vi "探头数据读取.vi"(11 "编号":string) -> ()   [LabVIEW 2016, in "斯坦道多参数.lvlib"]
panel:
  out "运行状态":u16(ring) items=["空闲", "水样测试", "标样核查"]
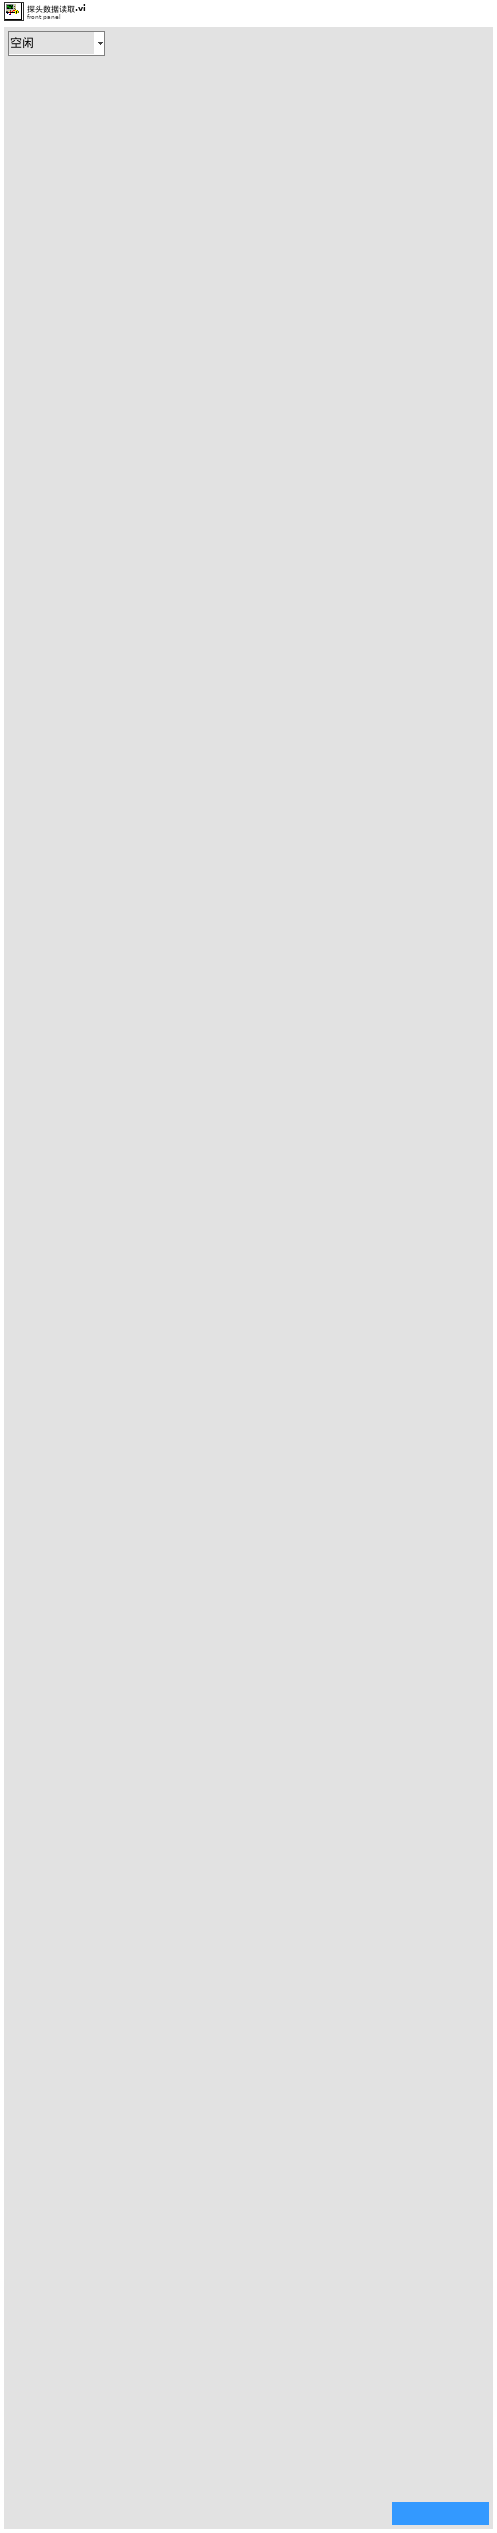
[diagram p1: front panel]
types:
  T1 = enum16{"pH", "DO", "Cond", "Turb", "ORP", "叶绿素a", "藻密度", "COD"}
  T2 = cluster{"温度测量值":sgl, "测量值":sgl, "温度偏移修正值":sgl, "信号值":sgl}
  T3 = cluster{"温度测量值":sgl, "DO%":sgl, "DOmg/L":sgl, "温度偏移修正值":sgl}
  T4 = cluster{"CH":u16, "监测值":dbl, "温度偏移修正值":sgl, "信号值":sgl}
  T5 = cluster{"pH探头选择":u16, "DO探头选择":u16, "电导率探头选择":u16, "浊度探头选择":u16, "叶绿素a探头选择":u16, "蓝绿藻探头选择":u16, "orp探头选择":u16, "COD探头选择":u16}
  T6 = cluster{"电极状态标志":u16, "电极型号标志":u16, "酸碱度测量值":sgl, "温度测量值":sgl, "酸碱度信号值":sgl, "温度信号值":sgl, "酸碱度偏移修正值":sgl, "温度偏移修正值":sgl, "手动温度补偿值":sgl, "酸碱度电极零点":sgl, "酸碱度电极斜率":sgl, "第1点标准值记录":sgl, "第1点信号值记录":sgl, "第1点温度值记录":sgl, "第2点标准值记录":sgl, "第2点信号值记录":sgl, "第2点温度值记录":sgl, "命令滤波设定":u16, "温度模式":enum16{"ATC", "MTC"}, "生产批次":u16, "电极序号":u16, "串口地址":u16, "串口波特率":enum16{"9600", "19200", "115200"}, "串口校验位":enum16{"NONE", "ODD", "EVEN"}, "串口停止位":enum16{"1bit", "2bit"}, "第一点标准值":sgl, "第二点标准值":sgl}
  T7 = cluster{"报警码":u16, "pH数值":sgl, "0X0003_NC":sgl, "温度数据":sgl, "pH原始信号 mv":sgl, "0X0009_NC":string, "产品名称":string, "序列号":string, "硬件版本":string, "软件版本":string, "通讯地址":u16, "波特率":u16, "设备类型":u16, "0X0026_NC":string, "第一点原始数据":sgl, "第一点校准数据":sgl, "第二点原始数据":sgl, "第二点校准数据":sgl, "探头校准命令":u16, "温度校准参数":sgl, "温度校准命令":u16}
  T8 = cluster{"电极状态标志":u16, "电极型号标志":u16, "电导率测量值":sgl, "温度测量值":sgl, "电导率信号值":sgl, "温度信号值":sgl, "温度补偿系数":sgl, "电导率偏移修正值":sgl, "温度偏移修正值":sgl, "手动温度补偿值":sgl, "电导率电极零点":sgl, "电导率电极斜率":sgl, "命令滤波设定":u16, "温度模式":enum16{"ATC", "MTC"}, "生产批次":u16, "电极序号":u16, "串口地址":u16, "串口波特率":enum16{"9600", "19200", "115200"}, "串口校验位":enum16{"NONE", "ODD", "EVEN"}, "串口停止位":enum16{"1bit", "2bit"}, "第一点标准值":sgl, "第二点标准值":sgl}
  T9 = cluster{"报警码":u16, "电导率数据（uS/cm）":sgl, "0x0003 NC":sgl, "温度数据":sgl, "电导率原始信号电阻":sgl, "当前量程":u16, "温度补偿系数":sgl, "0X0009_NC":string, "产品名称":string, "序列号":string, "硬件版本":string, "软件版本":string, "通讯地址":u16, "波特率":u16, "设备类型":u16, "0X0026_NC":string, "第一点原始数据":sgl, "第一点校准数据":sgl, "0X0035_NC":sgl, "0X0037_NC":sgl, "探头校准命令":u16, "温度校准参数":sgl, "温度校准命令":u16}
  T10 = cluster{"电极状态标志":u16, "电极型号标志":u16, "溶解氧测量值":sgl, "温度测量值":sgl, "溶解氧饱和度值":sgl, "盐度补偿值":sgl, "大气压补偿值":sgl, "溶解氧偏移修正值":sgl, "温度偏移修正值":sgl, "手动温度补偿值":sgl, "溶解氧电极零点":sgl, "溶解氧电极斜率":sgl, "第1点标准值记录":sgl, "第1点信号值记录":sgl, "第1点温度值记录":sgl, "第2点标准值记录":sgl, "第2点信号值记录":sgl, "第2点温度值记录":sgl, "命令滤波设定":u16, "温度模式":enum16{"ATC", "MTC"}, "生产批次":u16, "电极序号":u16, "串口地址":u16, "串口波特率":enum16{"9600", "19200", "115200"}, "串口校验位":enum16{"NONE", "ODD", "EVEN"}, "串口停止位":enum16{"1bit", "2bit"}, "第一点标准值":sgl, "第二点标准值":sgl}
  T11 = cluster{"报警码":u16, "溶解氧数值（mg/L）":sgl, "溶解氧数据（%）":sgl, "温度数据":sgl, "溶解氧原始信号 nA":sgl, "大气压力":sgl, "盐度":sgl, "0X0009_NC":string, "产品名称":string, "序列号":string, "硬件版本":string, "软件版本":string, "通讯地址":u16, "波特率":u16, "设备类型":u16, "0X0026_NC":string, "第一点原始数据":sgl, "0X0033 NC":sgl, "第二点原始数据":sgl, "0X0037 NC":sgl, "探头校准命令":u16, "温度校准参数":sgl, "温度校准命令":u16}
  T12 = cluster{"电极状态标志":u16, "电极型号标志":u16, "浊度测量值":sgl, "温度测量值":sgl, "浊度信号值":sgl, "浊度偏移修正值":sgl, "温度偏移修正值":sgl, "手动温度补偿值":sgl, "浊度电极零点":sgl, "浊度电极斜率":sgl, "第1点标准值记录":sgl, "第1点信号值记录":sgl, "第1点温度值记录":sgl, "第2点标准值记录":sgl, "第2点信号值记录":sgl, "第2点温度值记录":sgl, "命令滤波设定":u16, "温度模式":enum16{"ATC", "MTC"}, "生产批次":u16, "电极序号":u16, "串口地址":u16, "串口波特率":enum16{"9600", "19200", "115200"}, "串口校验位":enum16{"NONE", "ODD", "EVEN"}, "串口停止位":enum16{"1bit", "2bit"}, "第一点标准值":sgl, "第二点标准值":sgl, "第三点标准值":sgl}
  T13 = cluster{"报警码":u16, "浊度数值 NTU":sgl, "温度数据":sgl, "原始光强数值":u16, "量程":u16, "平均次数":u16, "清扫模式":u16, "清扫次数":u16, "清扫间隔分钟":u16, "0X000B_NC":string, "产品名称":string, "序列号":string, "硬件版本":string, "软件版本":string, "通讯地址":u16, "波特率":u16, "设备类型":u16, "0X0026_NC":string, "校准量程":u16, "第一点原始光强":u16, "第一点校准数据":sgl, "第二点原始光强":u16, "第二点校准数据":sgl, "第三点原始光强":u16, "第三点校准数据":sgl, "探头校准命令":u16, "温度校准参数":sgl, "温度校准命令":u16}
  T14 = cluster{"电极状态标志":u16, "电极型号标志":u16, "测量值":sgl, "温度测量值":sgl, "信号值":sgl, "温度信号值":sgl, "000AH_NC":sgl, "偏移修正值":sgl, "温度偏移修正值":sgl, "手动温度补偿值":sgl, "命令滤波设定":u16, "温度模式":enum16{"ATC", "MTC"}, "生产批次":u16, "传感器序号":u16, "串口地址":u16, "串口波特率":enum16{"9600", "19200", "115200"}, "串口校验位":enum16{"NONE", "ODD", "EVEN"}, "串口停止位":enum16{"1bit", "2bit"}}
  T15 = cluster{"报警码":u16, "叶绿素a":sgl, "温度数据":sgl, "原始光强数值":u16, "量程":u16, "平均次数":u16, "清扫模式":u16, "清扫次数":u16, "清扫间隔分钟":u16, "0X000B_NC":string, "产品名称":string, "序列号":string, "硬件版本":string, "软件版本":string, "通讯地址":u16, "波特率":u16, "设备类型":u16, "0X0026_NC":string, "校准量程":u16, "第一点原始光强":u16, "第一点校准数据":sgl, "第二点原始光强":u16, "第二点校准数据":sgl, "第三点原始光强":u16, "第三点校准数据":sgl, "探头校准命令":u16, "温度校准参数":sgl, "温度校准命令":u16}
  T16 = cluster{"报警码":u16, "蓝绿藻":sgl, "温度数据":sgl, "原始光强数值":u16, "0X0006_NC":u16, "平均次数":u16, "清扫模式":u16, "清扫次数":u16, "清扫间隔分钟":u16, "0X000B_NC":string, "产品名称":string, "序列号":string, "硬件版本":string, "软件版本":string, "通讯地址":u16, "波特率":u16, "设备类型":u16, "0X0026_NC":string, "0X0030_NC":u16, "第一点原始光强":u16, "第一点校准数据":sgl, "第二点原始光强":u16, "第二点校准数据":sgl, "第三点原始光强":u16, "第三点校准数据":sgl, "探头校准命令":u16, "温度校准参数":sgl, "温度校准命令":u16}
  T17 = cluster{"电极状态标志":u16, "电极型号标志":u16, "COD测量值":sgl, "浊度测量值":sgl, "COD信号值":sgl, "浊度信号值":sgl, "温度测量值":sgl, "COD偏移修正值":sgl, "浊度偏移修正值":sgl, "COD水样校正值":sgl, "温度偏移修正值":sgl, "COD零点系数":sgl, "COD斜率系数":sgl, "浊度零点系数":sgl, "浊度斜率系数":sgl, "COD测值K值":sgl, "浊度测值K值":sgl, "浊度补偿COD系数值":sgl, "COD温度补偿系数值 ":sgl, "测量周期":u16, "清洗周期":u16, "命令寄存器":u16, "数字滤波设定":u16, "温度模式":enum16{"AUTO", "OFF"}, "生产批次":u16, "电极序号":u16, "串口地址":u16, "串口波特率":enum16{"9600", "19200", "115200"}, "串口校验位":enum16{"NONE", "ODD", "EVEN"}, "串口停止位":enum16{"1bit", "2bit"}, "第一点校正指令":u16, "第一点标准值":sgl, "第二点校正指令":u16, "第二点标准值":sgl, "第三点校正指令":u16, "第三点标准值":sgl, "COD吸光度":sgl, "浊度吸光度":sgl, "温度信号值":sgl}
  T18 = enum16{"pH", "DO", "Cond", "Turb", "ORP", "叶绿素a", "藻密度", "COD"}[]
  T19 = cluster{"ph":bool, "DO":bool, "Cond":bool, "Turb":bool, "叶绿素a":bool, "藻密度":bool, "ORP":bool, "COD":bool}
  T20 = cluster{"ph":bool, "DO":bool, "Cond":bool, "Turb":bool, "叶绿素a":bool, "藻密度":bool, "ORP":bool, "cod":bool}
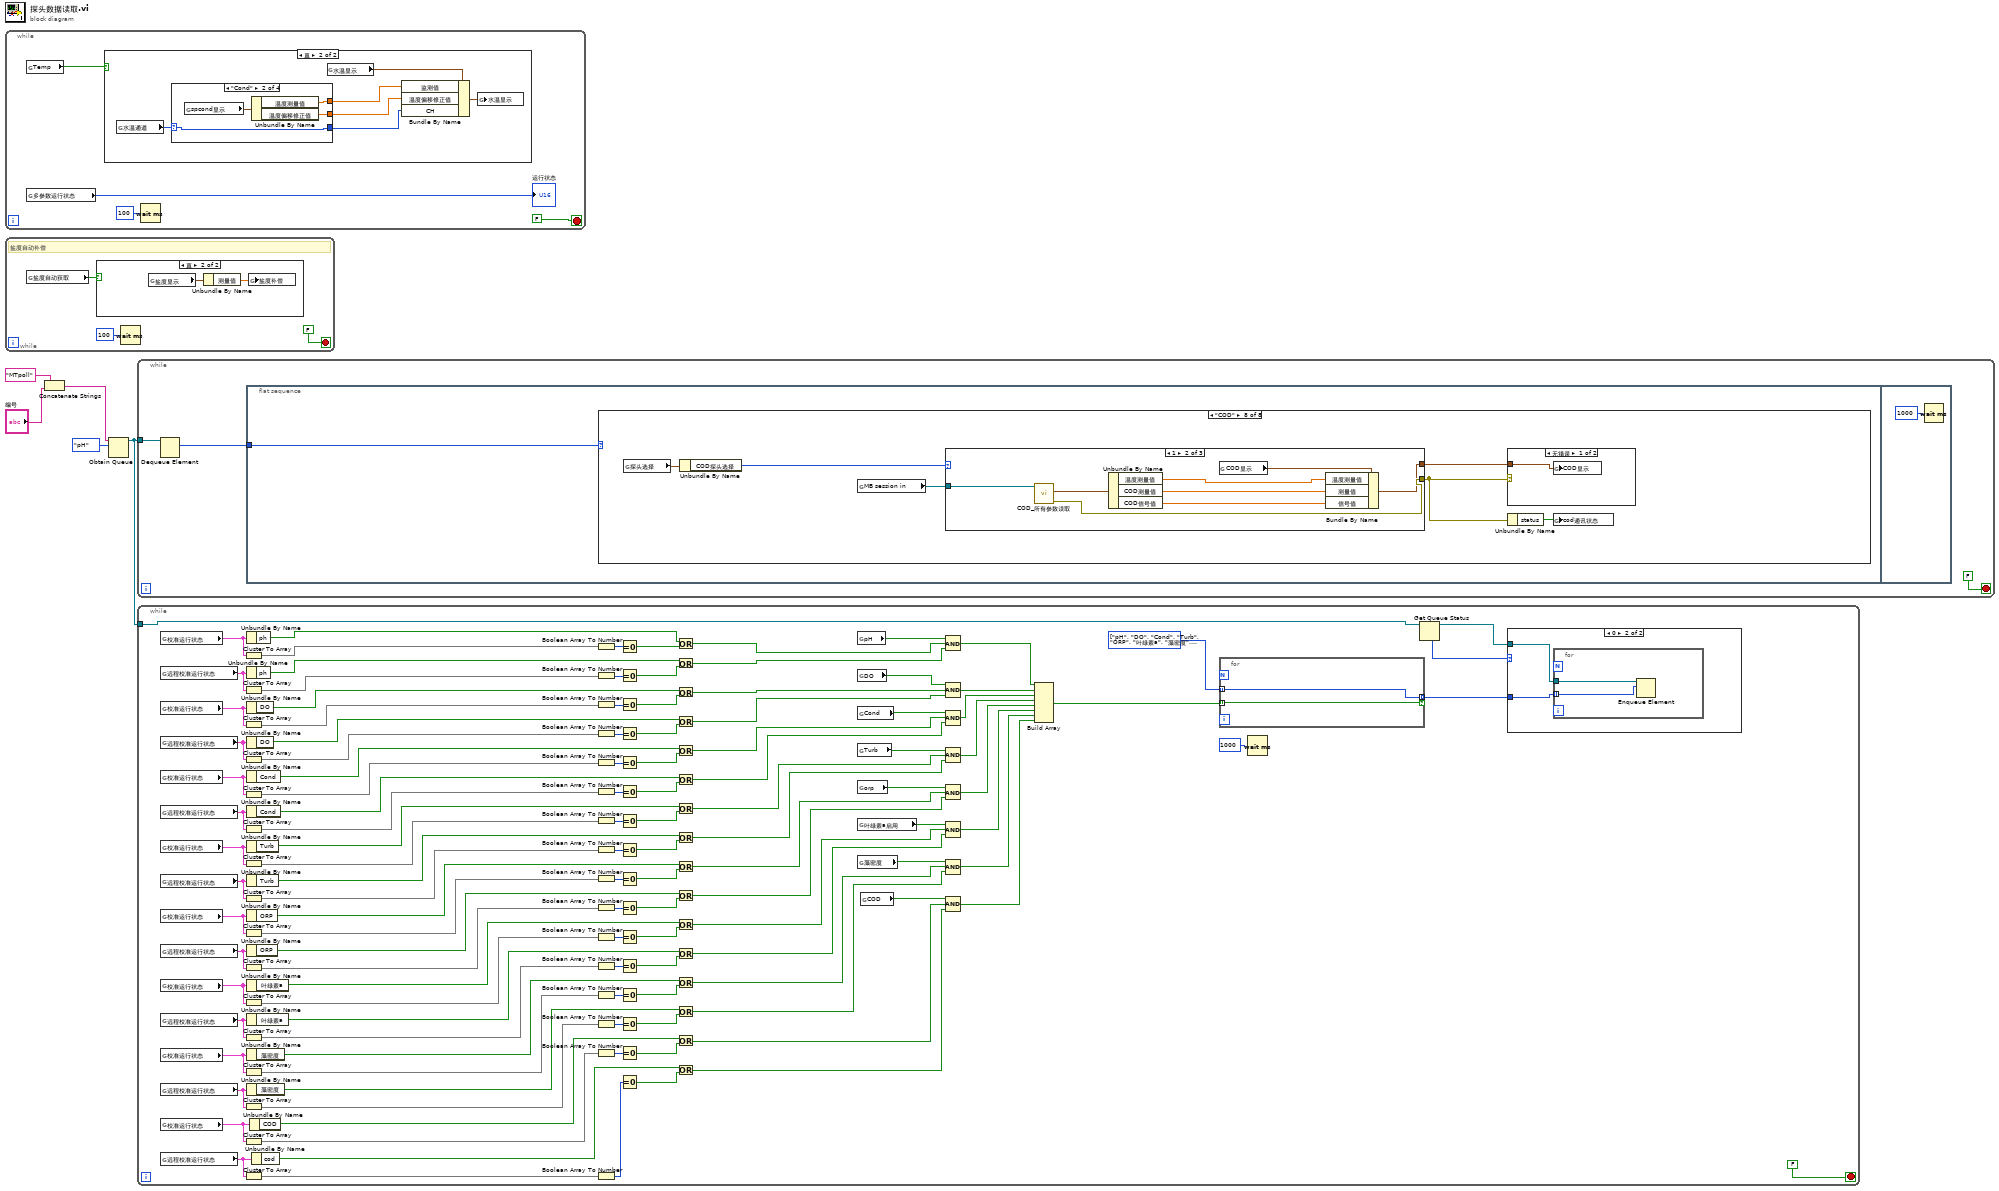
[diagram p0: block diagram]
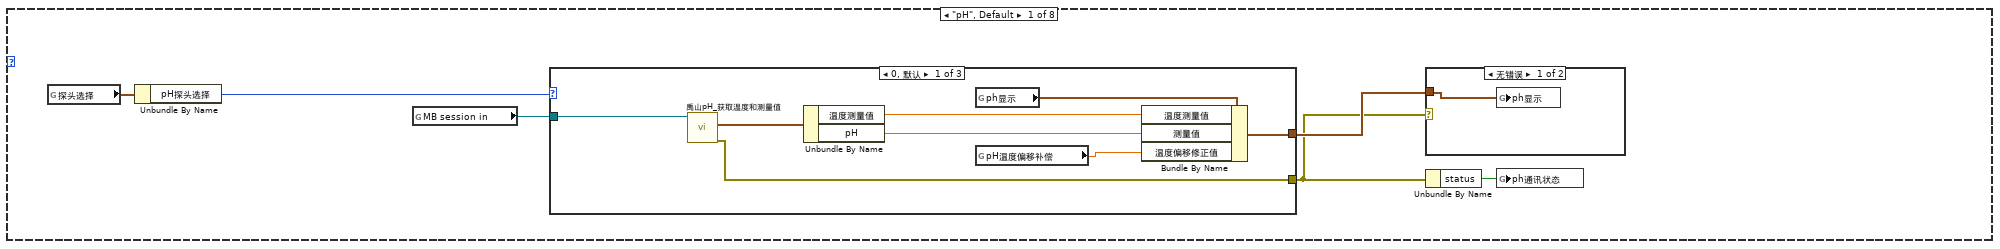
[diagram p3: hidden frame]
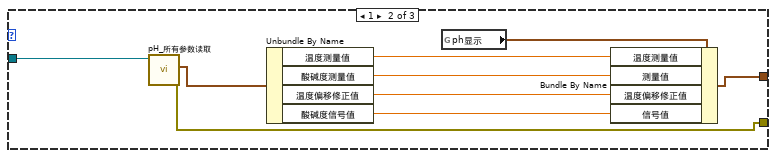
[diagram p4: hidden frame]
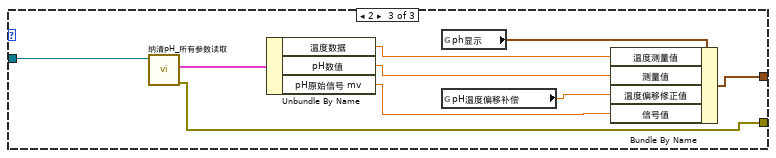
[diagram p5: hidden frame]
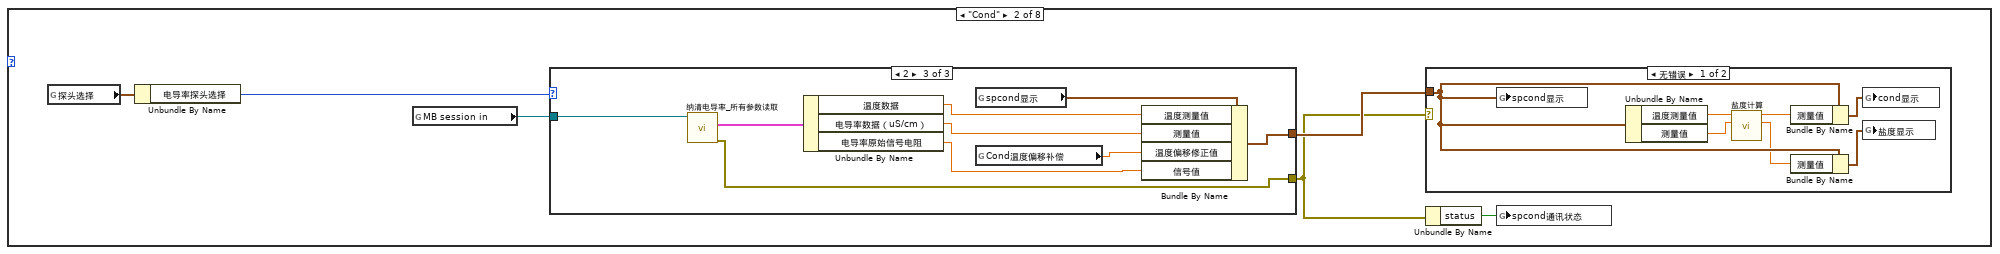
[diagram p7: hidden frame]
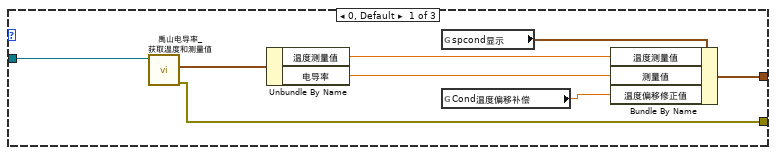
[diagram p8: hidden frame]
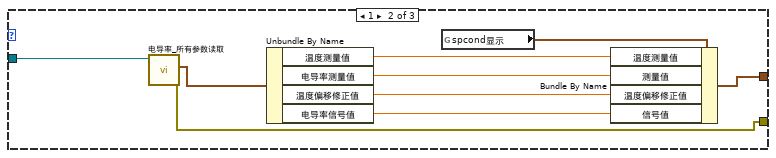
[diagram p9: hidden frame]
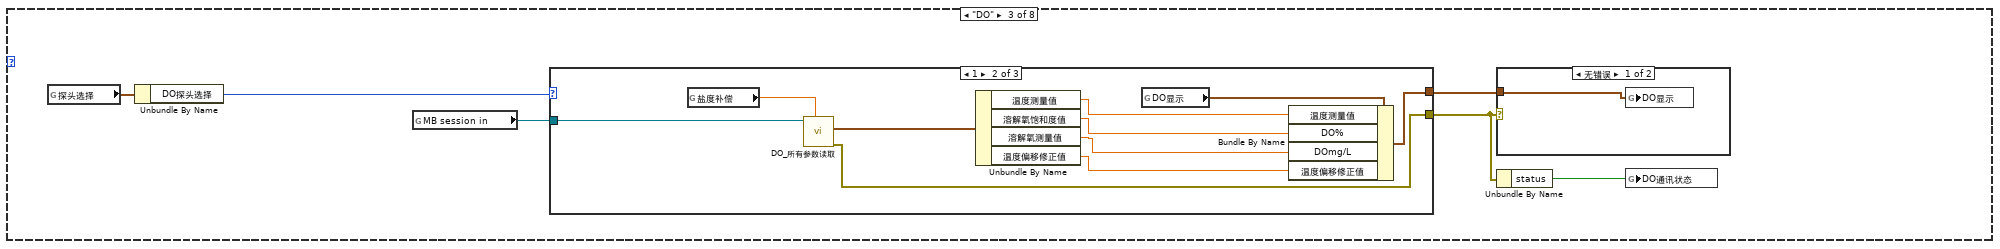
[diagram p11: hidden frame]
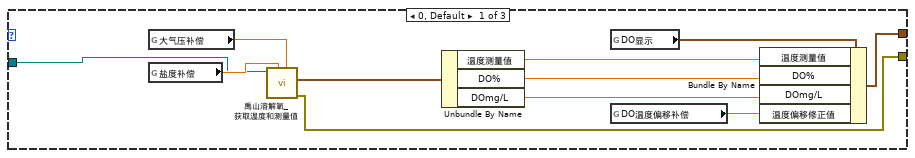
[diagram p12: hidden frame]
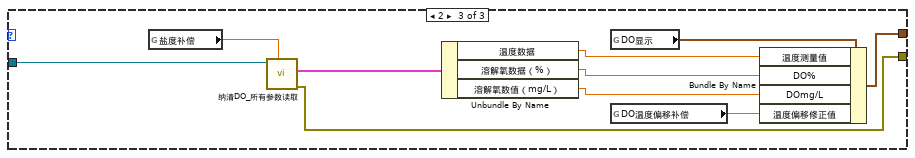
[diagram p13: hidden frame]
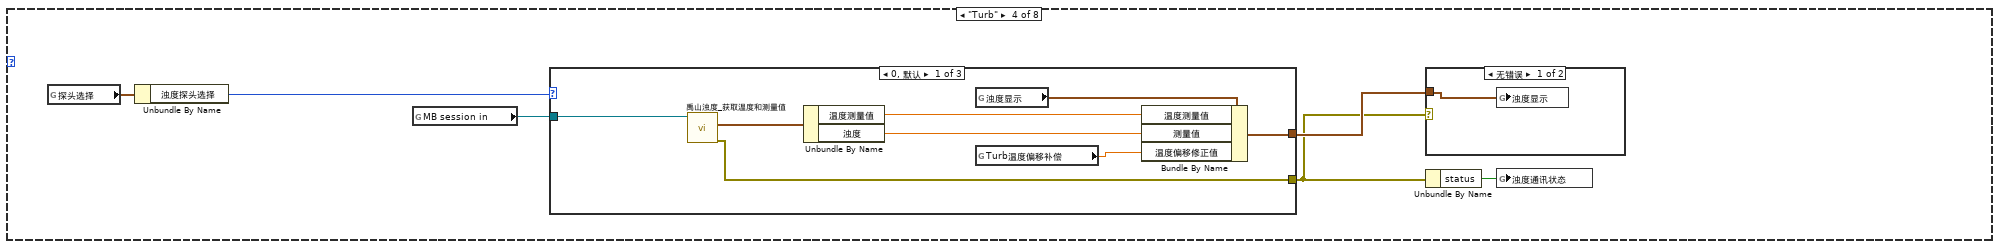
[diagram p15: hidden frame]
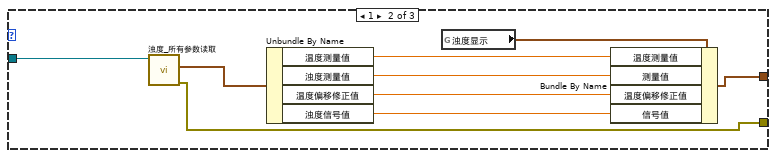
[diagram p16: hidden frame]
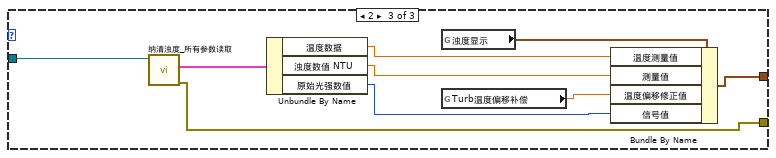
[diagram p17: hidden frame]
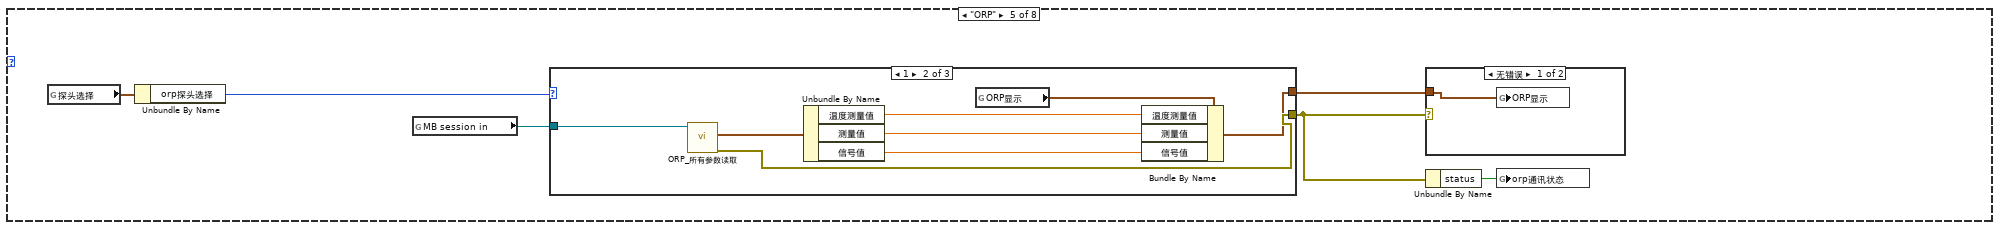
[diagram p19: hidden frame]
diagram:
  n1 = while {
    stop <- FALSE stop-if-true
    n2 = global read "断电保存变量.vi" "Temp"() -> (w7:bool)
    n3 = global read "多参数全局变量.vi" "多参数运行状态"() -> (→"运行状态":u16)
    n4 = case shown="真" w7 {
      frame False {
      }
      frame True {
        n5 = global read "断电保存变量.vi" "水温通道"() -> (w15:enum16{"pH", "Cond", "DO", "Turb"})
        n6 = case shown="\"Cond\"" w15 {
          selector: w15 -> [w19 w23 w27 w31]
          tunnel: [w19 w23 w27 w31] -> w14
          tunnel: [w17 w20 w24 w28] -> w13
          tunnel: [w18 w21 w25 w29] -> w12
          frame "pH", Default {
            n7 = global read "多参数全局变量.vi" "ph显示"() -> (w16:T2)
            n8 = Unbundle By Name(w16) -> ("温度测量值"=w18:sgl, "温度偏移修正值"=w17:sgl)
          }
          frame "Cond" {
            n9 = global read "多参数全局变量.vi" "spcond显示"() -> (w22:T2)
            n10 = Unbundle By Name(w22) -> ("温度测量值"=w21:sgl, "温度偏移修正值"=w20:sgl)
          }
          frame "DO" {
            n11 = global read "多参数全局变量.vi" "DO显示"() -> (w26:T3)
            n12 = Unbundle By Name(w26) -> ("温度测量值"=w25:sgl, "温度偏移修正值"=w24:sgl)
          }
          frame "Turb" {
            n13 = global read "多参数全局变量.vi" "浊度显示"() -> (w30:T2)
            n14 = Unbundle By Name(w30) -> ("温度测量值"=w29:sgl, "温度偏移修正值"=w28:sgl)
          }
        }
        n15 = global read "多参数全局变量.vi" "水温显示"() -> (w10:T4)
        n16 = Bundle By Name(cluster=w10, "监测值"=w12, "温度偏移修正值"=w13, "CH"=w14) -> (w11:T4)
        n17 = global write "多参数全局变量.vi" "水温显示"(w11) -> ()
      }
    }
    n18 = Wait (ms)(milliseconds to wait=u32 100 ("等待时间（毫秒）")) -> ()  [unwired: 1 out]
  }
  n19 = while {
    stop <- FALSE stop-if-true
    # "盐度自动补偿"
    n20 = global read "断电保存变量.vi" "盐度自动获取"() -> (w33:bool)
    n21 = case shown="真" w33 {
      frame False {
      }
      frame True {
        n22 = global read "多参数全局变量.vi" "盐度显示"() -> (w36:T2)
        n23 = Unbundle By Name(w36) -> ("测量值"=w35:sgl)
        n24 = global write "断电保存变量.vi" "盐度补偿"(w35) -> ()
      }
    }
    n25 = Wait (ms)(milliseconds to wait=u32 100 ("等待时间（毫秒）")) -> ()  [unwired: 1 out]
  }
  n26 = Concatenate Strings("MTpoll" ("名称（未命名）"), "编号") -> (w3:string)
  n27 = Obtain Queue(name (unnamed)=w3, element data type=T1."pH" ("枚举")) -> (queue out=w1:refnum<queue>)  [unwired: 3 in, 2 out]
  n28 = while {
    tunnel: w1 -> [w39]
    stop <- FALSE stop-if-true
    n29 = Dequeue Element(queue=w39) -> (element=w38:T1)  [unwired: 2 in, 3 out]
    n30 = flat-sequence {
      tunnel: w38 -> [w40]
      frame #0 {
        n31 = case shown="\"COD\"" w40 {
          frame "pH", Default {
            n32 = global read "断电保存变量.vi" "探头选择"() -> (w46:T5)
            n33 = Unbundle By Name(w46) -> ("pH探头选择"=w45:u16)
            n34 = global read "多参数全局变量.vi" "MB session in"() -> (w44:refnum<class "MB_Master.lvclass">)
            n35 = case shown="0, 默认" w45 {
              tunnel: w44 -> [w54 w63 w70]
              tunnel: [w53 w62 w68] -> w42
              tunnel: [w51 w59 w71] -> w43
              frame 0, Default {
                n36 = call "禹山pH_获取温度和测量值.vi"("MB session in"=w54) -> ("error out"=w53:errorcluster, "输出值"=w50:cluster{"温度测量值":sgl, "ORP":sgl, "pH":sgl})  [unwired: 8 in, 1 out]
                n37 = Unbundle By Name(w50) -> ("温度测量值"=w49:sgl, "pH"=w48:sgl)
                n38 = global read "多参数全局变量.vi" "ph显示"() -> (w52:T2)
                n39 = global read "断电保存变量.vi" "pH温度偏移补偿"() -> (w47:dbl)
                n40 = Bundle By Name(cluster=w52, "温度测量值"=w49, "测量值"=w48, "温度偏移修正值"=w47) -> (w51:T2)
              }
              frame 1 {
                n41 = call "pH_所有参数读取.vi"("MB session in"=w63) -> ("error out"=w62:errorcluster, "输出值"=w61:T6)  [unwired: 8 in, 1 out]
                n42 = Unbundle By Name(w61) -> ("温度测量值"=w56:sgl, "酸碱度测量值"=w57:sgl, "温度偏移修正值"=w58:sgl, "酸碱度信号值"=w55:sgl)
                n43 = global read "多参数全局变量.vi" "ph显示"() -> (w60:T2)
                n44 = Bundle By Name(cluster=w60, "温度测量值"=w56, "测量值"=w57, "温度偏移修正值"=w58, "信号值"=w55) -> (w59:T2)
              }
              frame 2 {
                n45 = call "纳清pH_所有参数读取.vi"("MB session in"=w70) -> ("error out"=w68:errorcluster, "输出值"=w69:T7)  [unwired: 8 in, 1 out]
                n46 = Unbundle By Name(w69) -> ("温度数据"=w67:sgl, "pH数值"=w66:sgl, "pH原始信号 mv"=w64:sgl)
                n47 = global read "多参数全局变量.vi" "ph显示"() -> (w72:T2)
                n48 = global read "断电保存变量.vi" "pH温度偏移补偿"() -> (w65:dbl)
                n49 = Bundle By Name(cluster=w72, "温度测量值"=w67, "测量值"=w66, "温度偏移修正值"=w65, "信号值"=w64) -> (w71:T2)
              }
            }
            n50 = case shown="无错误" w42 {
              tunnel: w43 -> [w73 _]
              frame No Error {
                n51 = global write "多参数全局变量.vi" "ph显示"(w73) -> ()
              }
              frame Error {
              }
            }
            n52 = Unbundle By Name(w42) -> ("status"=w41:bool)
            n53 = global write "多参数全局变量.vi" "ph通讯状态"(w41) -> ()
          }
          frame "Cond" {
            n54 = global read "断电保存变量.vi" "探头选择"() -> (w79:T5)
            n55 = Unbundle By Name(w79) -> ("电导率探头选择"=w78:u16)
            n56 = global read "多参数全局变量.vi" "MB session in"() -> (w76:refnum<class "MB_Master.lvclass">)
            n57 = case shown="2" w78 {
              tunnel: w76 -> [w87 w96 w101]
              tunnel: [w81 w94 w104] -> w77
              tunnel: [w86 w93 w99] -> w75
              frame 0, Default {
                n58 = call "禹山电导率_获取温度和测量值.vi"("MB session in"=w87) -> ("error out"=w86:errorcluster, "输出值"=w84:cluster{"温度测量值":sgl, "电导率":sgl, "错误标志":u16})  [unwired: 8 in, 1 out]
                n59 = Unbundle By Name(w84) -> ("温度测量值"=w83:sgl, "电导率"=w82:sgl)
                n60 = global read "多参数全局变量.vi" "spcond显示"() -> (w85:T2)
                n61 = global read "断电保存变量.vi" "Cond温度偏移补偿"() -> (w80:dbl)
                n62 = Bundle By Name(cluster=w85, "温度测量值"=w83, "测量值"=w82, "温度偏移修正值"=w80) -> (w81:T2)
              }
              frame 1 {
                n63 = call "电导率_所有参数读取.vi"("MB session in"=w96) -> ("error out"=w93:errorcluster, "输出值"=w92:T8)  [unwired: 8 in, 1 out]
                n64 = Unbundle By Name(w92) -> ("温度测量值"=w91:sgl, "电导率测量值"=w90:sgl, "温度偏移修正值"=w89:sgl, "电导率信号值"=w88:sgl)
                n65 = global read "多参数全局变量.vi" "spcond显示"() -> (w95:T2)
                n66 = Bundle By Name(cluster=w95, "温度测量值"=w91, "测量值"=w90, "温度偏移修正值"=w89, "信号值"=w88) -> (w94:T2)
              }
              frame 2 {
                n67 = call "纳清电导率_所有参数读取.vi"("MB session in"=w101) -> ("error out"=w99:errorcluster, "输出值"=w100:T9)  [unwired: 8 in, 1 out]
                n68 = Unbundle By Name(w100) -> ("温度数据"=w103:sgl, "电导率数据（uS/cm）"=w102:sgl, "电导率原始信号电阻"=w97:sgl)
                n69 = global read "多参数全局变量.vi" "spcond显示"() -> (w105:T2)
                n70 = global read "断电保存变量.vi" "Cond温度偏移补偿"() -> (w98:dbl)
                n71 = Bundle By Name(cluster=w105, "温度测量值"=w103, "测量值"=w102, "温度偏移修正值"=w98, "信号值"=w97) -> (w104:T2)
              }
            }
            n72 = case shown="无错误" w75 {
              tunnel: w77 -> [w107 _]
              frame No Error {
                n73 = global write "多参数全局变量.vi" "spcond显示"(w107) -> ()
                n74 = Unbundle By Name(w107) -> ("温度测量值"=w112:sgl, "测量值"=w111:sgl)
                n75 = call "盐度计算.vi"("spCond"=w111, "Temp"=w112) -> ("saltresult"=w106:dbl, "cond"=w110:dbl)  [unwired: 8 in]
                n76 = Bundle By Name(cluster=w107, "测量值"=w110) -> (w109:T2)
                n77 = Bundle By Name(cluster=w107, "测量值"=w106) -> (w108:T2)
                n78 = global write "多参数全局变量.vi" "cond显示"(w109) -> ()
                n79 = global write "多参数全局变量.vi" "盐度显示"(w108) -> ()
              }
              frame Error {
              }
            }
            n80 = Unbundle By Name(w75) -> ("status"=w74:bool)
            n81 = global write "多参数全局变量.vi" "spcond通讯状态"(w74) -> ()
          }
          frame "DO" {
            n82 = global read "断电保存变量.vi" "探头选择"() -> (w118:T5)
            n83 = Unbundle By Name(w118) -> ("DO探头选择"=w117:u16)
            n84 = global read "多参数全局变量.vi" "MB session in"() -> (w115:refnum<class "MB_Master.lvclass">)
            n85 = case shown="1" w117 {
              tunnel: w115 -> [w127 w139 w144]
              tunnel: [w125 w137 w148] -> w116
              tunnel: [w121 w132 w142] -> w114
              frame 0, Default {
                n86 = global read "断电保存变量.vi" "大气压补偿"() -> (w128:dbl)
                n87 = global read "断电保存变量.vi" "盐度补偿"() -> (w129:dbl)
                n88 = call "禹山溶解氧_获取温度和测量值.vi"("大气压补偿"=w128, "盐度补偿"=w129, "MB session in"=w127) -> ("error out"=w121:errorcluster, "输出值"=w119:cluster{"温度测量值":sgl, "DO%":sgl, "DOmg/L":sgl})  [unwired: 6 in, 1 out]
                n89 = Unbundle By Name(w119) -> ("温度测量值"=w124:sgl, "DO%"=w123:sgl, "DOmg/L"=w122:sgl)
                n90 = global read "多参数全局变量.vi" "DO显示"() -> (w126:T3)
                n91 = global read "断电保存变量.vi" "DO温度偏移补偿"() -> (w120:dbl)
                n92 = Bundle By Name(cluster=w126, "温度测量值"=w124, "DO%"=w123, "DOmg/L"=w122, "温度偏移修正值"=w120) -> (w125:T3)
              }
              frame 1 {
                n93 = global read "断电保存变量.vi" "盐度补偿"() -> (w130:dbl)
                n94 = call "DO_所有参数读取.vi"("盐度补偿"=w130, "MB session in"=w139) -> ("error out"=w132:errorcluster, "输出值"=w136:T10)  [unwired: 7 in, 1 out]
                n95 = Unbundle By Name(w136) -> ("温度测量值"=w133:sgl, "溶解氧饱和度值"=w134:sgl, "溶解氧测量值"=w135:sgl, "温度偏移修正值"=w131:sgl)
                n96 = global read "多参数全局变量.vi" "DO显示"() -> (w138:T3)
                n97 = Bundle By Name(cluster=w138, "温度测量值"=w133, "DO%"=w134, "DOmg/L"=w135, "温度偏移修正值"=w131) -> (w137:T3)
              }
              frame 2 {
                n98 = global read "断电保存变量.vi" "盐度补偿"() -> (w140:dbl)
                n99 = call "纳清DO_所有参数读取.vi"("盐度补偿"=w140, "MB session in"=w144) -> ("error out"=w142:errorcluster, "输出值"=w143:T11)  [unwired: 7 in, 1 out]
                n100 = Unbundle By Name(w143) -> ("温度数据"=w145:sgl, "溶解氧数据（%）"=w146:sgl, "溶解氧数值（mg/L）"=w147:sgl)
                n101 = global read "多参数全局变量.vi" "DO显示"() -> (w149:T3)
                n102 = global read "断电保存变量.vi" "DO温度偏移补偿"() -> (w141:dbl)
                n103 = Bundle By Name(cluster=w149, "温度测量值"=w145, "DO%"=w146, "DOmg/L"=w147, "温度偏移修正值"=w141) -> (w148:T3)
              }
            }
            n104 = case shown="无错误" w114 {
              tunnel: w116 -> [w150 _]
              frame No Error {
                n105 = global write "多参数全局变量.vi" "DO显示"(w150) -> ()
              }
              frame Error {
              }
            }
            n106 = Unbundle By Name(w114) -> ("status"=w113:bool)
            n107 = global write "多参数全局变量.vi" "DO通讯状态"(w113) -> ()
          }
          frame "Turb" {
            n108 = global read "断电保存变量.vi" "探头选择"() -> (w156:T5)
            n109 = Unbundle By Name(w156) -> ("浊度探头选择"=w155:u16)
            n110 = global read "多参数全局变量.vi" "MB session in"() -> (w153:refnum<class "MB_Master.lvclass">)
            n111 = case shown="0, 默认" w155 {
              tunnel: w153 -> [w164 w173 w178]
              tunnel: [w162 w168 w179] -> w154
              tunnel: [w161 w167 w177] -> w152
              frame 0, Default {
                n112 = call "禹山浊度_获取温度和测量值.vi"("MB session in"=w164) -> ("error out"=w161:errorcluster, "输出值"=w160:cluster{"温度测量值":sgl, "浊度":sgl})  [unwired: 8 in, 1 out]
                n113 = Unbundle By Name(w160) -> ("温度测量值"=w159:sgl, "浊度"=w158:sgl)
                n114 = global read "多参数全局变量.vi" "浊度显示"() -> (w163:T2)
                n115 = global read "断电保存变量.vi" "Turb温度偏移补偿"() -> (w157:dbl)
                n116 = Bundle By Name(cluster=w163, "温度测量值"=w159, "测量值"=w158, "温度偏移修正值"=w157) -> (w162:T2)
              }
              frame 1 {
                n117 = call "浊度_所有参数读取.vi"("MB session in"=w173) -> ("error out"=w167:errorcluster, "输出值"=w172:T12)  [unwired: 8 in, 1 out]
                n118 = Unbundle By Name(w172) -> ("温度测量值"=w170:sgl, "浊度测量值"=w169:sgl, "温度偏移修正值"=w166:sgl, "浊度信号值"=w165:sgl)
                n119 = global read "多参数全局变量.vi" "浊度显示"() -> (w171:T2)
                n120 = Bundle By Name(cluster=w171, "温度测量值"=w170, "测量值"=w169, "温度偏移修正值"=w166, "信号值"=w165) -> (w168:T2)
              }
              frame 2 {
                n121 = call "纳清浊度_所有参数读取.vi"("MB session in"=w178) -> ("error out"=w177:errorcluster, "输出值"=w176:T13)  [unwired: 8 in, 1 out]
                n122 = Unbundle By Name(w176) -> ("温度数据"=w181:sgl, "浊度数值 NTU"=w180:sgl, "原始光强数值"=w174:u16)
                n123 = global read "多参数全局变量.vi" "浊度显示"() -> (w182:T2)
                n124 = global read "断电保存变量.vi" "Turb温度偏移补偿"() -> (w175:dbl)
                n125 = Bundle By Name(cluster=w182, "温度测量值"=w181, "测量值"=w180, "温度偏移修正值"=w175, "信号值"=w174) -> (w179:T2)
              }
            }
            n126 = case shown="无错误" w152 {
              tunnel: w154 -> [w183 _]
              frame No Error {
                n127 = global write "多参数全局变量.vi" "浊度显示"(w183) -> ()
              }
              frame Error {
              }
            }
            n128 = Unbundle By Name(w152) -> ("status"=w151:bool)
            n129 = global write "多参数全局变量.vi" "浊度通讯状态"(w151) -> ()
          }
          frame "ORP" {
            n130 = global read "断电保存变量.vi" "探头选择"() -> (w188:T5)
            n131 = Unbundle By Name(w188) -> ("orp探头选择"=w187:u16)
            n132 = global read "多参数全局变量.vi" "MB session in"() -> (w186:refnum<class "MB_Master.lvclass">)
            n133 = case shown="1" w187 {
              tunnel: [_ w192 _] -> w185
              tunnel: w186 -> [_ w197 _]
              tunnel: [_ w190 _] -> w189
              frame 0, Default {
              }
              frame 1 {
                n134 = call "ORP_所有参数读取.vi"("MB session in"=w197) -> ("error out"=w192:errorcluster, "输出值"=w194:T14)  [unwired: 8 in, 1 out]
                n135 = Unbundle By Name(w194) -> ("温度测量值"=w195:sgl, "测量值"=w196:sgl, "信号值"=w191:sgl)
                n136 = global read "多参数全局变量.vi" "ORP显示"() -> (w193:T2)
                n137 = Bundle By Name(cluster=w193, "温度测量值"=w195, "测量值"=w196, "信号值"=w191) -> (w190:T2)
              }
              frame 2 {
              }
            }
            n138 = case shown="无错误" w185 {
              tunnel: w189 -> [w198 _]
              frame No Error {
                n139 = global write "多参数全局变量.vi" "ORP显示"(w198) -> ()
              }
              frame Error {
              }
            }
            n140 = Unbundle By Name(w185) -> ("status"=w184:bool)
            n141 = global write "多参数全局变量.vi" "orp通讯状态"(w184) -> ()
          }
          frame "叶绿素a" {
            n142 = global read "断电保存变量.vi" "探头选择"() -> (w203:T5)
            n143 = Unbundle By Name(w203) -> ("叶绿素a探头选择"=w202:u16)
            n144 = global read "多参数全局变量.vi" "MB session in"() -> (w201:refnum<class "MB_Master.lvclass">)
            n145 = case shown="2" w202 {
              tunnel: [w211 _ w217] -> w200
              tunnel: w201 -> [w210 _ w219]
              tunnel: [w208 _ w216] -> w204
              frame 0, Default {
                n146 = call "叶绿素a_获取温度和叶绿素值.vi"("MB session in"=w210) -> ("error out"=w211:errorcluster, "输出值"=w207:cluster{"温度测量值":sgl, "叶绿素测量值":sgl, "错误标志":u16})  [unwired: 8 in, 1 out]
                n147 = Unbundle By Name(w207) -> ("温度测量值"=w205:sgl, "叶绿素测量值"=w206:sgl)
                n148 = global read "多参数全局变量.vi" "叶绿素a显示"() -> (w209:T2)
                n149 = Bundle By Name(cluster=w209, "温度测量值"=w205, "测量值"=w206) -> (w208:T2)
              }
              frame 1 {
              }
              frame 2 {
                n150 = call "纳清叶绿素a_所有参数读取.vi"("MB session in"=w219) -> ("error out"=w217:errorcluster, "输出值"=w215:T15)  [unwired: 8 in, 1 out]
                n151 = Unbundle By Name(w215) -> ("温度数据"=w213:sgl, "叶绿素a"=w214:sgl, "原始光强数值"=w212:u16)
                n152 = global read "多参数全局变量.vi" "叶绿素a显示"() -> (w218:T2)
                n153 = Bundle By Name(cluster=w218, "温度测量值"=w213, "测量值"=w214, "信号值"=w212) -> (w216:T2)
              }
            }
            n154 = case shown="无错误" w200 {
              tunnel: w204 -> [w220 _]
              frame No Error {
                n155 = global write "多参数全局变量.vi" "叶绿素a显示"(w220) -> ()
              }
              frame Error {
              }
            }
            n156 = Unbundle By Name(w200) -> ("status"=w199:bool)
            n157 = global write "多参数全局变量.vi" "叶绿素a通讯状态"(w199) -> ()
          }
          frame "藻密度" {
            n158 = global read "断电保存变量.vi" "探头选择"() -> (w225:T5)
            n159 = Unbundle By Name(w225) -> ("蓝绿藻探头选择"=w224:u16)
            n160 = global read "多参数全局变量.vi" "MB session in"() -> (w223:refnum<class "MB_Master.lvclass">)
            n161 = case shown="2" w224 {
              tunnel: [_ _ w232] -> w222
              tunnel: w223 -> [_ _ w234]
              tunnel: [_ _ w231] -> w226
              frame 0, Default {
              }
              frame 1 {
              }
              frame 2 {
                n162 = call "纳清蓝绿藻_所有参数读取.vi"("MB session in"=w234) -> ("error out"=w232:errorcluster, "输出值"=w230:T16)  [unwired: 8 in, 1 out]
                n163 = Unbundle By Name(w230) -> ("温度数据"=w229:sgl, "蓝绿藻"=w228:sgl, "原始光强数值"=w227:u16)
                n164 = global read "多参数全局变量.vi" "藻密度显示"() -> (w233:T2)
                n165 = Bundle By Name(cluster=w233, "温度测量值"=w229, "测量值"=w228, "信号值"=w227) -> (w231:T2)
              }
            }
            n166 = case shown="无错误" w222 {
              tunnel: w226 -> [w235 _]
              frame No Error {
                n167 = global write "多参数全局变量.vi" "藻密度显示"(w235) -> ()
              }
              frame Error {
              }
            }
            n168 = Unbundle By Name(w222) -> ("status"=w221:bool)
            n169 = global write "多参数全局变量.vi" "藻密度通讯状态"(w221) -> ()
          }
          frame "COD" {
            n170 = global read "断电保存变量.vi" "探头选择"() -> (w240:T5)
            n171 = Unbundle By Name(w240) -> ("COD探头选择"=w239:u16)
            n172 = global read "多参数全局变量.vi" "MB session in"() -> (w238:refnum<class "MB_Master.lvclass">)
            n173 = case shown="1" w239 {
              tunnel: [_ w247 _] -> w237
              tunnel: w238 -> [_ w249 _]
              tunnel: [_ w246 _] -> w241
              frame 0, Default {
              }
              frame 1 {
                n174 = call "COD_所有参数读取.vi"("MB session in"=w249) -> ("error out"=w247:errorcluster, "输出值"=w245:T17)  [unwired: 8 in, 1 out]
                n175 = Unbundle By Name(w245) -> ("温度测量值"=w244:sgl, "COD测量值"=w243:sgl, "COD信号值"=w242:sgl)
                n176 = global read "多参数全局变量.vi" "COD显示"() -> (w248:T2)
                n177 = Bundle By Name(cluster=w248, "温度测量值"=w244, "测量值"=w243, "信号值"=w242) -> (w246:T2)
              }
              frame 2 {
              }
            }
            n178 = case shown="无错误" w237 {
              tunnel: w241 -> [w250 _]
              frame No Error {
                n179 = global write "多参数全局变量.vi" "COD显示"(w250) -> ()
              }
              frame Error {
              }
            }
            n180 = Unbundle By Name(w237) -> ("status"=w236:bool)
            n181 = global write "多参数全局变量.vi" "cod通讯状态"(w236) -> ()
          }
        }
      }
      frame #1 {
        n182 = Wait (ms)(milliseconds to wait=u32 1000 ("等待时间（毫秒）")) -> ()  [unwired: 1 out]
      }
    }
  }
  n183 = while {
    tunnel: w1 -> [w371]
    stop <- FALSE stop-if-true
    w270 = T18 [enum."pH", enum."DO", enum."Cond", enum."Turb", enum."ORP", enum."叶绿素a", enum."藻密度", enum."COD"] items=["pH", "DO", "Cond", "Turb", "ORP", "叶绿素a", "藻密度", "COD"]
    n184 = global read "多参数全局变量.vi" "校准运行状态"() -> (w357:T19)
    n185 = global read "多参数全局变量.vi" "远程校准运行状态"() -> (w368:T20)
    n186 = global read "多参数全局变量.vi" "校准运行状态"() -> (w331:T19)
    n187 = global read "多参数全局变量.vi" "远程校准运行状态"() -> (w342:T20)
    n188 = global read "多参数全局变量.vi" "校准运行状态"() -> (w356:T19)
    n189 = global read "多参数全局变量.vi" "远程校准运行状态"() -> (w345:T20)
    n190 = global read "多参数全局变量.vi" "校准运行状态"() -> (w318:T19)
    n191 = global read "多参数全局变量.vi" "远程校准运行状态"() -> (w329:T20)
    n192 = global read "多参数全局变量.vi" "校准运行状态"() -> (w305:T19)
    n193 = global read "多参数全局变量.vi" "远程校准运行状态"() -> (w316:T20)
    n194 = global read "多参数全局变量.vi" "校准运行状态"() -> (w304:T19)
    n195 = global read "多参数全局变量.vi" "远程校准运行状态"() -> (w293:T20)
    n196 = global read "多参数全局变量.vi" "校准运行状态"() -> (w279:T19)
    n197 = global read "多参数全局变量.vi" "远程校准运行状态"() -> (w290:T20)
    n198 = global read "多参数全局变量.vi" "校准运行状态"() -> (w264:T19)
    n199 = global read "多参数全局变量.vi" "远程校准运行状态"() -> (w257:T20)
    n200 = Cluster To Array(cluster=w357) -> (array=w362:bool[])
    n201 = Cluster To Array(cluster=w368) -> (array=w364:bool[])
    n202 = Cluster To Array(cluster=w331) -> (array=w336:bool[])
    n203 = Cluster To Array(cluster=w342) -> (array=w338:bool[])
    n204 = Cluster To Array(cluster=w356) -> (array=w351:bool[])
    n205 = Cluster To Array(cluster=w345) -> (array=w349:bool[])
    n206 = Cluster To Array(cluster=w318) -> (array=w323:bool[])
    n207 = Cluster To Array(cluster=w329) -> (array=w325:bool[])
    n208 = Cluster To Array(cluster=w305) -> (array=w310:bool[])
    n209 = Cluster To Array(cluster=w316) -> (array=w312:bool[])
    n210 = Cluster To Array(cluster=w304) -> (array=w299:bool[])
    n211 = Cluster To Array(cluster=w293) -> (array=w297:bool[])
    n212 = Cluster To Array(cluster=w279) -> (array=w284:bool[])
    n213 = Cluster To Array(cluster=w290) -> (array=w286:bool[])
    n214 = Cluster To Array(cluster=w264) -> (array=w260:bool[])
    n215 = Cluster To Array(cluster=w257) -> (array=w256:bool[])
    n216 = Unbundle By Name(w357) -> ("ph"=w359:bool)
    n217 = Unbundle By Name(w368) -> ("ph"=w367:bool)
    n218 = Unbundle By Name(w331) -> ("DO"=w333:bool)
    n219 = Unbundle By Name(w342) -> ("DO"=w341:bool)
    n220 = Unbundle By Name(w356) -> ("Cond"=w354:bool)
    n221 = Unbundle By Name(w345) -> ("Cond"=w346:bool)
    n222 = Unbundle By Name(w318) -> ("Turb"=w320:bool)
    n223 = Unbundle By Name(w329) -> ("Turb"=w328:bool)
    n224 = Unbundle By Name(w305) -> ("ORP"=w307:bool)
    n225 = Unbundle By Name(w316) -> ("ORP"=w315:bool)
    n226 = Unbundle By Name(w304) -> ("叶绿素a"=w302:bool)
    n227 = Unbundle By Name(w293) -> ("叶绿素a"=w294:bool)
    n228 = Unbundle By Name(w279) -> ("藻密度"=w281:bool)
    n229 = Unbundle By Name(w290) -> ("藻密度"=w289:bool)
    n230 = Unbundle By Name(w264) -> ("COD"=w263:bool)
    n231 = Unbundle By Name(w257) -> ("cod"=w258:bool)
    n232 = Boolean Array To Number(Boolean array=w362) -> (number=w361:u32)
    n233 = Boolean Array To Number(Boolean array=w364) -> (number=w365:u32)
    n234 = Boolean Array To Number(Boolean array=w336) -> (number=w335:u32)
    n235 = Boolean Array To Number(Boolean array=w338) -> (number=w339:u32)
    n236 = Boolean Array To Number(Boolean array=w351) -> (number=w352:u32)
    n237 = Boolean Array To Number(Boolean array=w349) -> (number=w348:u32)
    n238 = Boolean Array To Number(Boolean array=w323) -> (number=w322:u32)
    n239 = Boolean Array To Number(Boolean array=w325) -> (number=w326:u32)
    n240 = Boolean Array To Number(Boolean array=w310) -> (number=w309:u32)
    n241 = Boolean Array To Number(Boolean array=w312) -> (number=w313:u32)
    n242 = Boolean Array To Number(Boolean array=w299) -> (number=w300:u32)
    n243 = Boolean Array To Number(Boolean array=w297) -> (number=w296:u32)
    n244 = Boolean Array To Number(Boolean array=w284) -> (number=w283:u32)
    n245 = Boolean Array To Number(Boolean array=w286) -> (number=w287:u32)
    n246 = Boolean Array To Number(Boolean array=w260) -> (number=w261:u32)
    n247 = Boolean Array To Number(Boolean array=w256) -> (number=w255:u32)
    n248 = Equal To 0?(x=w361) -> (x = 0?=w360:bool)
    n249 = Equal To 0?(x=w365) -> (x = 0?=w366:bool)
    n250 = Equal To 0?(x=w335) -> (x = 0?=w334:bool)
    n251 = Equal To 0?(x=w339) -> (x = 0?=w340:bool)
    n252 = Equal To 0?(x=w352) -> (x = 0?=w353:bool)
    n253 = Equal To 0?(x=w348) -> (x = 0?=w347:bool)
    n254 = Equal To 0?(x=w322) -> (x = 0?=w321:bool)
    n255 = Equal To 0?(x=w326) -> (x = 0?=w327:bool)
    n256 = Equal To 0?(x=w309) -> (x = 0?=w308:bool)
    n257 = Equal To 0?(x=w313) -> (x = 0?=w314:bool)
    n258 = Equal To 0?(x=w300) -> (x = 0?=w301:bool)
    n259 = Equal To 0?(x=w296) -> (x = 0?=w295:bool)
    n260 = Equal To 0?(x=w283) -> (x = 0?=w282:bool)
    n261 = Equal To 0?(x=w287) -> (x = 0?=w288:bool)
    n262 = Equal To 0?(x=w261) -> (x = 0?=w262:bool)
    n263 = Equal To 0?(x=w255) -> (x = 0?=w259:bool)
    n264 = Or(x=w359, y=w360) -> (x .or. y?=w358:bool)
    n265 = Or(x=w367, y=w366) -> (x .or. y?=w369:bool)
    n266 = Or(x=w333, y=w334) -> (x .or. y?=w332:bool)
    n267 = Or(x=w341, y=w340) -> (x .or. y?=w343:bool)
    n268 = Or(x=w354, y=w353) -> (x .or. y?=w355:bool)
    n269 = Or(x=w346, y=w347) -> (x .or. y?=w344:bool)
    n270 = Or(x=w320, y=w321) -> (x .or. y?=w319:bool)
    n271 = Or(x=w328, y=w327) -> (x .or. y?=w330:bool)
    n272 = Or(x=w307, y=w308) -> (x .or. y?=w306:bool)
    n273 = Or(x=w315, y=w314) -> (x .or. y?=w317:bool)
    n274 = Or(x=w302, y=w301) -> (x .or. y?=w303:bool)
    n275 = Or(x=w294, y=w295) -> (x .or. y?=w292:bool)
    n276 = Or(x=w281, y=w282) -> (x .or. y?=w280:bool)
    n277 = Or(x=w289, y=w288) -> (x .or. y?=w291:bool)
    n278 = Or(x=w263, y=w262) -> (x .or. y?=w254:bool)
    n279 = Or(x=w258, y=w259) -> (x .or. y?=w253:bool)
    n280 = global read "断电保存变量.vi" "pH"() -> (w363:bool)
    n281 = global read "断电保存变量.vi" "DO"() -> (w337:bool)
    n282 = global read "断电保存变量.vi" "Cond"() -> (w350:bool)
    n283 = global read "断电保存变量.vi" "Turb"() -> (w324:bool)
    n284 = global read "断电保存变量.vi" "orp"() -> (w311:bool)
    n285 = global read "断电保存变量.vi" "叶绿素a启用"() -> (w298:bool)
    n286 = global read "断电保存变量.vi" "藻密度"() -> (w285:bool)
    n287 = global read "断电保存变量.vi" "COD"() -> (w265:bool)
    n288 = Compound Arithmetic op=AND ("复合运算")(w363, w358, w369) -> (w278:bool)
    n289 = Compound Arithmetic op=AND ("复合运算")(w337, w332, w343) -> (w277:bool)
    n290 = Compound Arithmetic op=AND ("复合运算")(w350, w355, w344) -> (w276:bool)
    n291 = Compound Arithmetic op=AND ("复合运算")(w324, w319, w330) -> (w275:bool)
    n292 = Compound Arithmetic op=AND ("复合运算")(w311, w306, w317) -> (w274:bool)
    n293 = Compound Arithmetic op=AND ("复合运算")(w298, w303, w292) -> (w273:bool)
    n294 = Compound Arithmetic op=AND ("复合运算")(w285, w280, w291) -> (w272:bool)
    n295 = Compound Arithmetic op=AND ("复合运算")(w265, w254, w253) -> (w252:bool)
    n296 = Build Array(w278, w277, w276, w275, w274, w273, w272, w252) -> (w271:bool[])
    n297 = for {
      tunnel: w271 -> [w376] mode=indexing
      tunnel: w270 -> [w377] mode=indexing
      tunnel: [w377] -> w269 mode=indexing if=w376
    }
    n298 = Wait (ms)(milliseconds to wait=u32 1000 ("等待时间（毫秒）")) -> ()  [unwired: 1 out]
    n299 = Get Queue Status(queue=w371) -> (queue out=w267:refnum<queue>, # elements in queue=w266:i32)  [unwired: 2 in, 6 out]
    n300 = case shown="0" w266 {
      tunnel: w269 -> [_ w373]
      tunnel: w267 -> [_ w372]
      frame Default {
      }
      frame 0 {
        n301 = for {
          tunnel: w372 -> [w375]
          tunnel: w373 -> [w374] mode=indexing
          n302 = Enqueue Element(queue=w375, element=w374) -> ()  [unwired: 2 in, 3 out]
        }
      }
    }
  }
